vi "MPM_Get_Each_Channel_Logdata.vi"(8 "error in (no error)":errorcluster, 9 "channelNumber":i32, 10 "moduleNumber":i32, 11 ".NET Reference in":refnum<k24>) -> (0 "error out":errorcluster, 2 "data out":sgl[](array[numeric]), 3 "Reference out":refnum<k24>)   [LabVIEW 2017]
uses:
  C:/Users/Ssantec_Test/Documents/Instrument_DLL_Sample_Labview_20250826_Ver1.5.0_x64/DLL/InstrumentDLL.dll
  DLL/InstrumentDLL.dll
panel:
  out "?":sgl[](array[numeric])
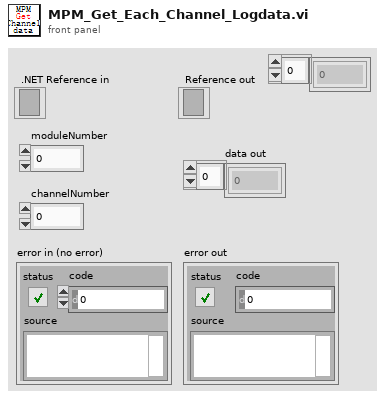
[diagram p1: front panel]
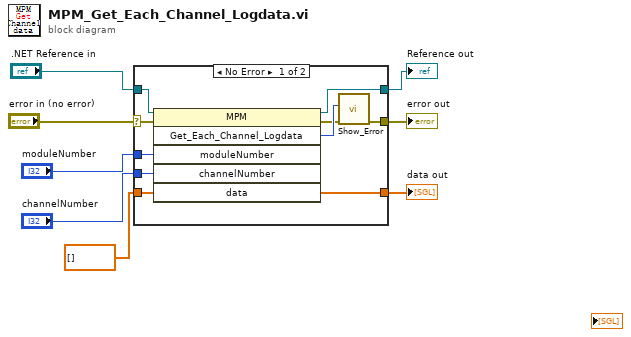
[diagram p0: block diagram]
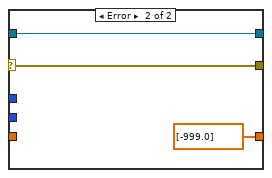
[diagram p2: hidden frame]
diagram:
  n1 = case shown="No Error" "error in (no error)" {
    selector: "error in (no error)" -> [w14 w20]
    tunnel: "channelNumber" -> [w18 _]
    tunnel: "moduleNumber" -> [w17 _]
    tunnel: ".NET Reference in" -> [w16 w21]
    tunnel: [w15 w21] -> w5
    tunnel: [w11 w20] -> w4
    tunnel: sgl[] [] ("data") -> [w10 _]
    tunnel: [w9 sgl[] [-999.0] ("data")] -> w1
    frame No Error {
      n2 = invoke class="MPM" method="Get_Each_Channel_Logdata"(reference=w16, error in=w14, "moduleNumber"=w17, "channelNumber"=w18, "data"=w10) -> (reference out=w15:refnum<k24>, error out=w12:errorcluster, "Get_Each_Channel_Logdata"=w13:i32, "data"=w9:sgl[])  [unwired: 1 in, 2 out]
      n3 = call "Show_Error.vi"("error in (no error)"=w12, "Error"=w13) -> ("error out"=w11:errorcluster)  [unwired: 9 in]
    }
    frame Error {
    }
  }
  "Reference out" <- w5
  "error out" <- w4
  "data out" <- w1
